vi "ThorLabs_Log_Write.vi"(0 "ThorLabs VISA":refnum<visa-resource-name>="ThorLabs", 5 "ThorLabs Log File":path=path "D:/WV_DIAL_Log_Files/TL.log", 11 "Error In":errorcluster) -> (4 "Log Entry":string[](array[string]), 15 "Error Out":errorcluster)   [LabVIEW 2012]
panel:
  in  "EXIT - No Write":bool
  in  "Write and EXIT":bool
  # "ThorLabs Log - Write"
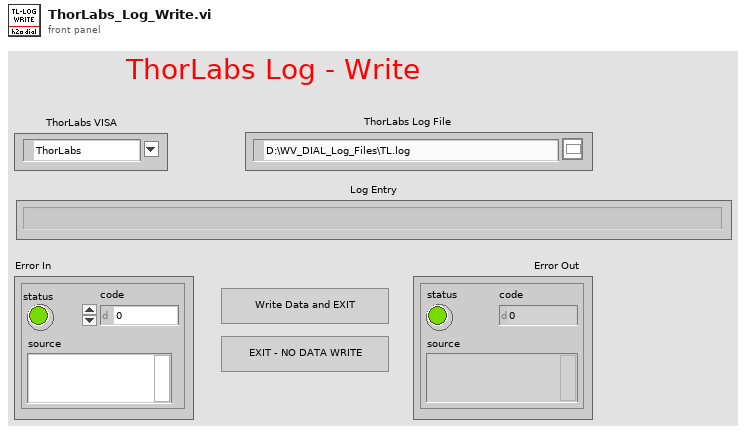
[diagram p1: front panel]
types:
  T1 = enum16{"open", "replace", "create", "open or create", "replace or create", "replace or create with confirmation"}
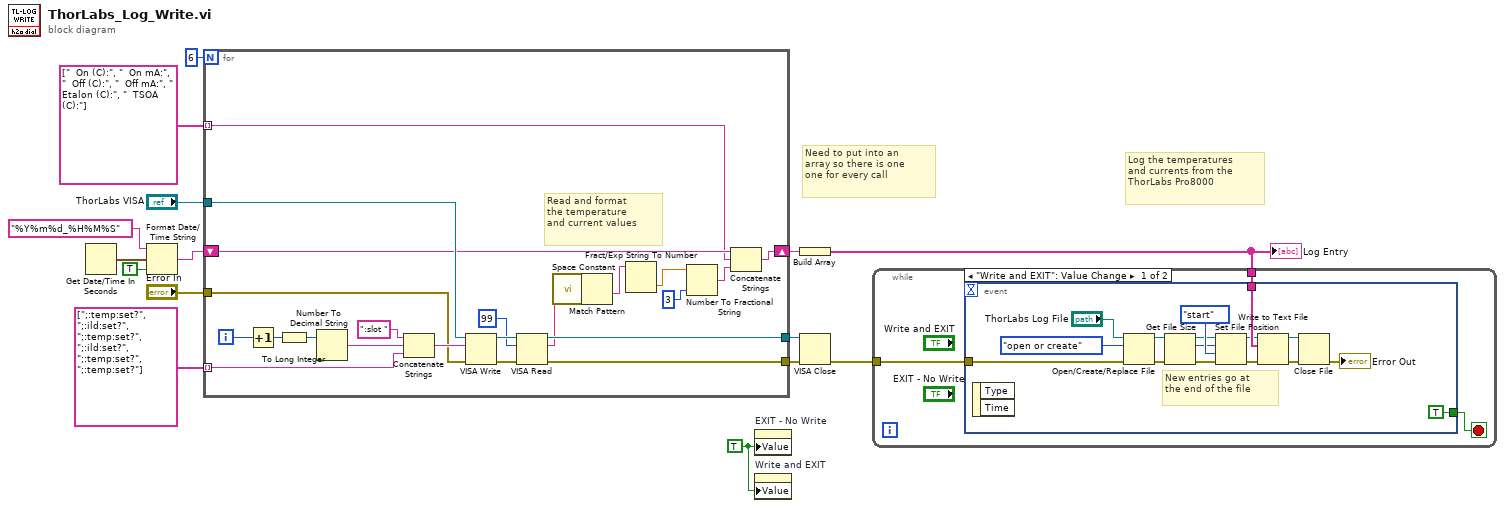
[diagram p0: block diagram]
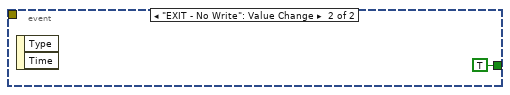
[diagram p2: hidden frame]
diagram:
  w1 = TRUE ("EXIT - No Write")
  # "Need to put into an\narray so there is one\none for every call"
  # "Log the temperatures\nand currents from the\nThorLabs Pro8000"
  n1 = Get Date/Time In Seconds() -> (seconds since 1Jan1904=w15:timestamp)
  n2 = Format Date/Time String(time format string (%c)="%Y%m%d_%H%M%S", seconds (now)=w15, UTC format=TRUE) -> (date/time string=w11:string)
  n3 = for {
    N: 6 -> [_]
    tunnel: "ThorLabs VISA" -> [w38]
    tunnel: [w37] -> w10
    tunnel: string[] [";:temp:set?", ";:ild:set?", ";:temp:set?", ";:ild:set?", ";:temp:set?", ";:temp:set?"] -> [w30] mode=indexing
    shift-right: [w26] -> w5
    shift-left: w11 -> [w28]
    tunnel: "Error In" -> [w29]
    tunnel: [w27] -> w9
    tunnel: string[] ["  On (C):", "  On mA:", "  Off (C):", "  Off mA:", "  Etalon (C):", "  TSOA (C):"] -> [w17] mode=indexing
    i -> [w36]
    # "Read and format\nthe temperature\nand current values"
    n4 = Increment(x=w36) -> (x+1=w31:i32)
    n5 = To Long Integer(number=w31) -> (32bit integer=w34:i32)
    n6 = Number To Decimal String(number=w34) -> (decimal integer string=w33:string)  [unwired: 1 in]
    n7 = Concatenate Strings(":slot ", w33, w30) -> (w35:string)
    n8 = VISA Write(VISA resource name=w38, write buffer=w35, error in (no error)=w29) -> (VISA resource name out=w20:refnum<visa-resource-name>, error out=w19:errorcluster)  [unwired: 1 out]
    n9 = VISA Read(VISA resource name=w20, byte count=u32 99, error in (no error)=w19) -> (VISA resource name out=w37:refnum<visa-resource-name>, read buffer=w21:string, error out=w27:errorcluster)  [unwired: 1 out]
    n10 = call <vilib>:"Space Constant.vi"() -> ("String"=w22:string)
    n11 = Match Pattern(string=w21, regular expression=w22) -> (after substring=w23:string)  [unwired: 1 in, 3 out]
    n12 = Fract/Exp String To Number(string=w23) -> (number=w24:dbl)  [unwired: 3 in, 1 out]
    n13 = Number To Fractional String(number=w24, precision (6)=i16 3) -> (F-format string=w16:string)  [unwired: 2 in]
    n14 = Concatenate Strings(w28, w17, w16) -> (w26:string)
  }
  n15 = property on="EXIT - No Write" class="Bool (strict)"("Value"=w1) -> ()  [unwired: 2 in, 2 out]
  n16 = property on="Write and EXIT" class="Bool (strict)"("Value"=w1) -> ()  [unwired: 2 in, 2 out]
  n17 = Build Array(w5) -> (w2:string[])
  "Log Entry" <- w2
  n18 = VISA Close(VISA resource name=w10, error in (no error)=w9) -> (error out=w7:errorcluster)
  n19 = while {
    tunnel: w7 -> [w41]
    tunnel: w2 -> [w40]
    stop <- w39 stop-if-true
    n20 = event shown="[0] \"Write and EXIT\": Value Change" {
      selector: _ -> [_ _]
      dyn-events: _ -> [_ _]
      timeout: _ -> [_ _]
      tunnel: w41 -> [w57 _]
      tunnel: w40 -> [w56 _]
      tunnel: [TRUE TRUE] -> w39
      event "Write and EXIT": Value Change {
        # "New entries go at\nthe end of the file"
        n21 = event-data() -> ()  [unwired: 1 in, 2 out]
        n22 = Open/Create/Replace File(file path (use dialog)="ThorLabs Log File", error in=w57, operation (0:open)=T1."open or create") -> (refnum out=w47:refnum<file>, error out=w44:errorcluster)  [unwired: 3 in, 1 out]
        n23 = Get File Size(file=w47, error in=w44) -> (refnum out=w48:refnum<file>, size (in bytes)=w43:i64, 0:w49:errorcluster)
        n24 = Set File Position(offset (in bytes) (0)=w43, refnum=w48, from (0:start)=enum16{"start", "end", "current"}."start", error in=w49) -> (refnum out=w51:refnum<file>, error out=w50:errorcluster)
        n25 = Write to Text File(file (use dialog)=w51, text=w56, error in=w50) -> (refnum out=w46:refnum<file>, error out=w45:errorcluster)  [unwired: 1 in, 1 out]
        n26 = Close File(refnum=w46, error in=w45) -> (error out=→"Error Out":errorcluster)  [unwired: 1 out]
      }
      event "EXIT - No Write": Value Change {
        n27 = event-data() -> ()  [unwired: 1 in, 2 out]
      }
    }
  }
